vi "闹钟（每秒）.vi"() -> (7 "TimeReached":bool)   [LabVIEW 2011]
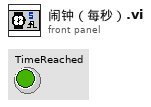
[diagram p1: front panel]
types:
  T1 = typedef "LVDateTimeRec.ctl" = cluster{"秒数的小数部分":dbl, "秒":i32, "分":i32, "时":i32, "日":i32, "月":i32, "年":i32, "天数（周）":i32, "天数（年）":i32, "DST":i32}
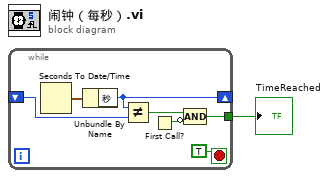
[diagram p0: block diagram]
diagram:
  n1 = while {
    shift-right: [w7] -> _
    shift-left: _ -> [w6]
    tunnel: [w3] -> w1
    stop <- TRUE stop-if-true
    n2 = Seconds To Date/Time() -> (date time rec=w8:T1)  [unwired: 2 in]
    n3 = Unbundle By Name(w8) -> ("秒"=w7:i32)
    n4 = Not Equal?(x=w7, y=w6) -> (x != y?=w4:bool)
    n5 = First Call?() -> (First Call?: T/F=w5:bool)
    n6 = Compound Arithmetic op=AND(w4, invert w5) -> (w3:bool)
  }
  "TimeReached" <- w1
